vi "Format Timestamp.vi"(10 "timestamp":timestamp, 11 "format string":string="%<%Y/%m/%d %H:%M:%S%3u>T") -> (3 "String":string)   [LabVIEW 2020, in "Communicable State Machine.lvlib"]
uses:
  Communicable State Machine.lvlib
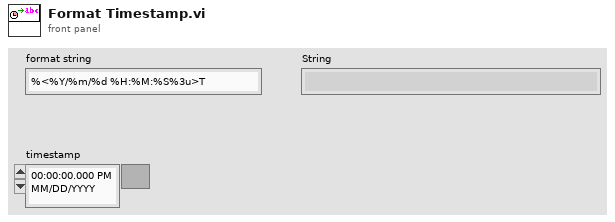
[diagram p1: front panel]
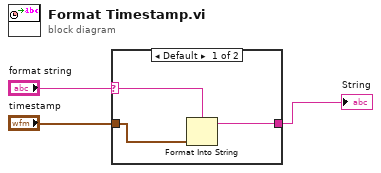
[diagram p0: block diagram]
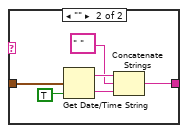
[diagram p2: hidden frame]
diagram:
  n1 = case shown="Default" "format string" {
    selector: "format string" -> [w5 _]
    tunnel: [w6 w10] -> w3
    tunnel: "timestamp" -> [w4 w7]
    frame Default {
      n2 = Format Into String(format string=w5, w4) -> (resulting string=w6:string)  [unwired: 2 in, 1 out]
    }
    frame "" {
      n3 = Get Date/Time String(seconds (now)=w7, want seconds? (F)=TRUE) -> (date string=w9:string, time string=w12:string)  [unwired: 1 in]
      n4 = Concatenate Strings(w9, " " ("string"), w12) -> (w10:string)
    }
  }
  "String" <- w3
